vi "OpenCVCam_LiveCapture.vi"(8 "ErrorIn":errorcluster, 10 "CmdData":variant, 11 "OpenCVCamIn":refnum<class>) -> (0 "ErrorOut":errorcluster, 2 "ReplyData":variant, 3 "OpenCVCamOut":refnum<class>, 4 "Exit":bool)   [LabVIEW 2021, in "OpenCVCam.lvclass"]
uses:
  OpenCVCam.lvclass
  OpenCVCam.lvclass/OpenCVCam.ctl
  OpenCVCam_UiCallBackEvents.ctl
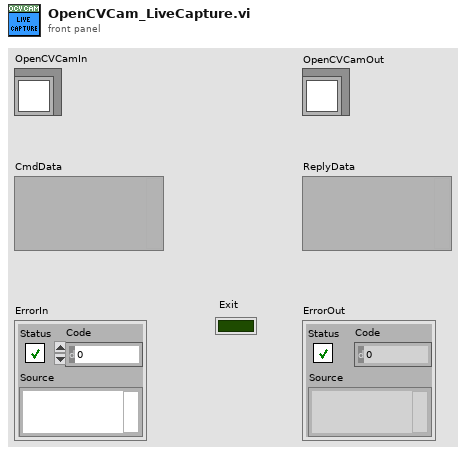
[diagram p1: front panel]
types:
  T1 = typedef "OpenCVCam.lvclass/OpenCVCam_UiCallBackEvents.ctl" = enum16{"Default", "PersistentDataUpdated", "NewPicture", "Worker 1: Do Something"}
  T2 = typedef "OpenCVCam.lvclass/State.ctl" = enum16{"Idle", "Initialized", "Acquiring"}
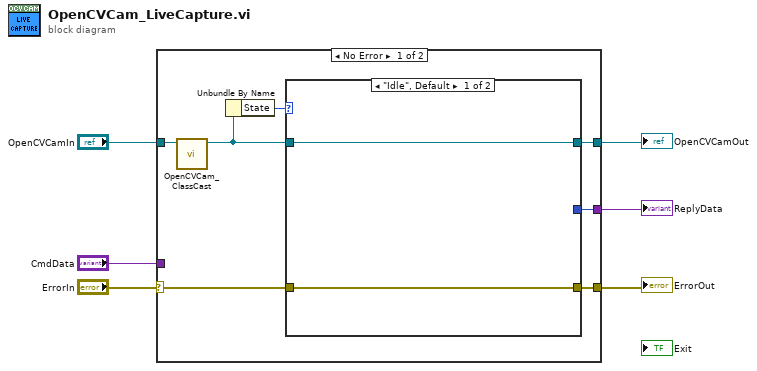
[diagram p0: block diagram]
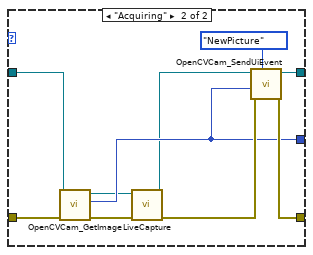
[diagram p2: hidden frame]
diagram:
  n1 = case shown="No Error" "ErrorIn" {
    selector: "ErrorIn" -> [w12 w28]
    tunnel: [w13 w28] -> w5
    tunnel: [w9 w27] -> w3
    tunnel: "CmdData" -> [_ w27]
    tunnel: "OpenCVCamIn" -> [w11 w26]
    tunnel: [w10 w26] -> w1
    frame No Error {
      n2 = call "OpenCVCam_ClassCast.vi"("OpenCVCamIn"=w11) -> ("OpenCVCamOut"=w8:refnum<class "OpenCVCam.lvclass">)  [unwired: 10 in]
      n3 = Unbundle By Name(w8) -> ("State"=w7:T2)
      n4 = case shown="\"Idle\", Default" w7 {
        tunnel: [w14 w21] -> w10
        tunnel: [w15 w25] -> w13
        tunnel: [_ w20] -> w9
        tunnel: w12 -> [w15 w24]
        tunnel: w8 -> [w14 w18]
        frame "Idle", Default {
        }
        frame "Acquiring" {
          n5 = call "OpenCVCam_GetImage.vi"("ErrorIn"=w24, "OpenCVCamIn"=w18) -> ("ErrorOut"=w23:errorcluster, "NewPicture"=w20:picture, "OpenCVCamOut"=w17:refnum<class "OpenCVCam.lvclass">)  [unwired: 7 in]
          n6 = call-dynamic "LiveCapture.vi"("ErrorIn"=w23, "OpenCVCamIn"=w17) -> ("ErrorOut"=w22:errorcluster, "OpenCVCamOut"=w16:refnum<class "OpenCVCam.lvclass">)  [unwired: 8 in]
          n7 = call "OpenCVCam_SendUiEvent.vi"("UiEventNames"=OpenCVCam_UiCallBackEvents."NewPicture", "ErrorIn"=w22, "Data"=w20, "OpenCVCamIn"=w16) -> ("ErrorOut"=w25:errorcluster, "OpenCVCamOut"=w21:refnum<class "OpenCVCam.lvclass">)  [unwired: 6 in]
        }
      }
    }
    frame Error {
    }
  }
  "ErrorOut" <- w5
  "OpenCVCamOut" <- w1
  "ReplyData" <- w3
